vi "Get Required Driver Types.vi"(8 "error in (no error)":errorcluster, 11 "Multi Instrument Msg in":refnum<class "Multi Instrument Msg.lvclass">) -> (0 "error out":errorcluster, 2 "Required Driver Types":T1[](array[typedef]), 3 "Multi Instrument Msg out":refnum<class "Multi Instrument Msg.lvclass">)   [LabVIEW 2020, in "Instrument Handler.lvlib" / "Multi Instrument Msg.lvclass"]
doc: "Get the Required Driver Types and count of each driver for execution of the Instrument Msg."
uses:
  Multi Instrument Msg.lvclass
  Ctl_RequiredInstrumentElement.ctl
  PPL/HDH.Actor Framework.Core.Instrument Driver.lvlibp/Instrument Driver/Instrument Driver.lvclass
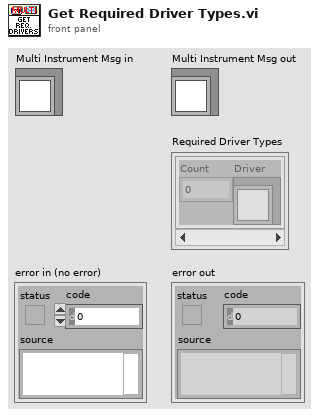
[diagram p1: front panel]
types:
  T1 = typedef "Instrument Handler.lvlib/Multi Instrument Msg.lvclass/Ctl_RequiredInstrumentElement.ctl" = cluster{"Count":i16, "Driver":refnum<class "Instrument Driver.lvclass">}
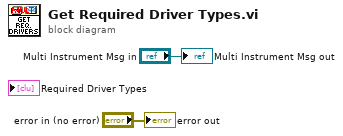
[diagram p0: block diagram]
diagram:
  "error out" <- "error in (no error)"
  "Multi Instrument Msg out" <- "Multi Instrument Msg in"
